vi "To Probe.vi"(8 "error in (no error)":errorcluster, 11 "NT Base in":refnum<class "NT Base.lvclass">) -> (0 "error out":errorcluster, 2 "Probe":T1, 3 "NT Base out":refnum<class "NT Base.lvclass">)   [LabVIEW 2020, in "PV Access.lvlib" / "PV Data.lvlib" / "NT Base.lvclass"]
uses:
  NT Base.lvclass
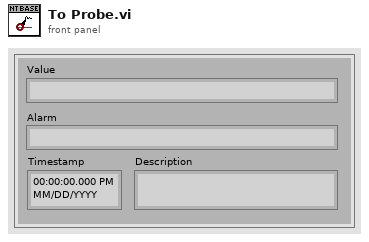
[diagram p1: front panel]
types:
  T1 = cluster{"Timestamp":timestamp, "Value":string, "Description":string, "Alarm":string}
  T2 = typedef "PV Access.lvlib/PV Data.lvlib/Alarm Severity.ctl" = enum32{"no", "minor", "major", "record", "invalid", "undefined", ""}
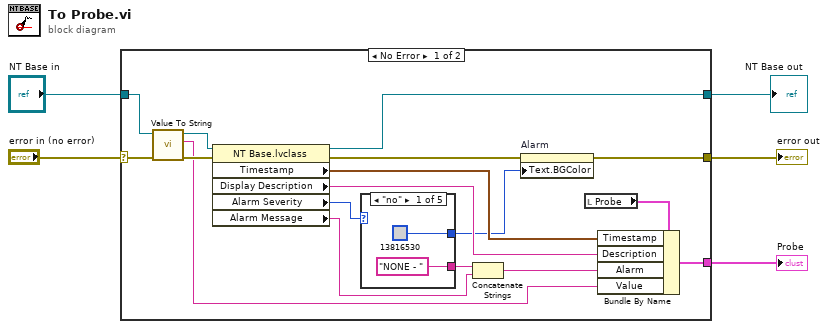
[diagram p0: block diagram]
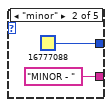
[diagram p2: hidden frame]
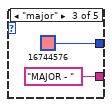
[diagram p3: hidden frame]
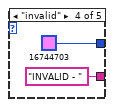
[diagram p4: hidden frame]
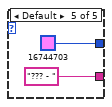
[diagram p5: hidden frame]
diagram:
  n1 = case shown="No Error" "error in (no error)" {
    selector: "error in (no error)" -> [w18 w34]
    tunnel: [w7 w34] -> w4
    tunnel: [w16 w33] -> w2
    tunnel: "NT Base in" -> [w17 w33]
    tunnel: [w22 _] -> w1
    frame No Error {
      n2 = call-dynamic "Value To String.vi"("error in (no error)"=w18, "NT Base in"=w17) -> ("error out"=w20:errorcluster, "string"=w13:string, "NT Base out"=w19:refnum<class "NT Base.lvclass">)  [unwired: 7 in]
      n3 = property class="NT Base.lvclass"(reference=w19, error in=w20) -> (reference out=w16:refnum<class "NT Base.lvclass">, error out=w8:errorcluster, "Timestamp"=w15:timestamp, "Display Description"=w14:string, "Alarm Severity"=w12:T2, "Alarm Message"=w10:string)
      n4 = case shown="\"no\"" w12 {
        tunnel: [u32 13816530 ("Text.BGColor") u32 16777088 ("Text.BGColor") u32 16744576 ("Text.BGColor") u32 16744703 ("Text.BGColor") u32 16744703 ("Text.BGColor")] -> w6
        tunnel: ["NONE - " "MINOR - " "MAJOR - " "INVALID - " "??? - "] -> w11
        frame "no" {
        }
        frame "minor" {
        }
        frame "major" {
        }
        frame "invalid" {
        }
        frame Default {
        }
      }
      n5 = Concatenate Strings(w11, w10) -> (w9:string)
      n6 = property on="Alarm" class="Str"(error in=w8, "Text.BGColor"=w6) -> (error out=w7:errorcluster)  [unwired: 1 in, 1 out]
      n7 = local read "Probe"() -> (w21:T1)
      n8 = Bundle By Name(cluster=w21, "Timestamp"=w15, "Description"=w14, "Alarm"=w9, "Value"=w13) -> (w22:T1)
    }
    frame Error {
    }
  }
  "error out" <- w4
  "NT Base out" <- w2
  "Probe" <- w1
